vi "Get Section.vi"(10 "Section":string, 11 "Dictionary in":refnum<class "Dictionary.lvclass">) -> (1 "Section out":refnum<class "Section.lvclass">, 2 "Found?":bool, 3 "Dictionary out":refnum<class "Dictionary.lvclass">)   [LabVIEW 2024, in "Electronic Datasheet.lvlib" / "Dictionary.lvclass"]
uses:
  Dictionary.lvclass
  OD Section/Section.lvclass
  Dictionary.lvclass/Dictionary.ctl
  Section Name/Section Name.lvclass
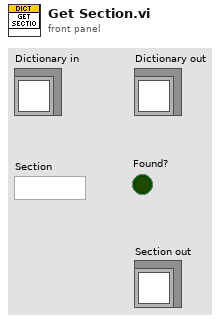
[diagram p1: front panel]
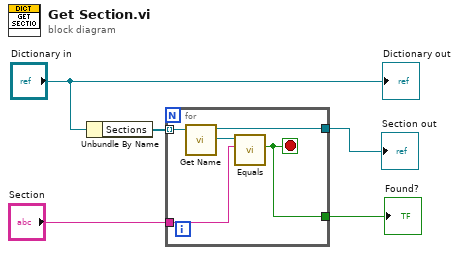
[diagram p0: block diagram]
diagram:
  n1 = Unbundle By Name("Dictionary in") -> ("Sections"=w4:refnum<class "Section.lvclass">[])
  n2 = for {
    tunnel: w4 -> [w10] mode=indexing
    tunnel: "Section" -> [w7]
    tunnel: [w9] -> w2
    tunnel: [w6] -> w1
    stop <- w6 stop-if-true
    n3 = call "Get Name.vi"("Object Entry in"=w10) -> ("Section Name"=w8:refnum<class "Section Name.lvclass">, "Object Entry out"=w9:refnum<class "Section.lvclass">)  [unwired: 9 in]
    n4 = call "Equals.vi"("String"=w7, "Section Name in"=w8) -> ("Equal?"=w6:bool)  [unwired: 8 in, 1 out]
  }
  "Section out" <- w2
  "Found?" <- w1
  "Dictionary out" <- "Dictionary in"
